vi "Periodic Tasks.vi"(8 "error in":errorcluster) -> ()   [LabVIEW 2020]
doc: "This VI runs in parallel to other tasks. It can contain as many user-defined periodic loops as you need. These can carry out PID or other sorts of timed response."
uses:
  <vilib>/Rock Robotics/WPI/ThirdParty/REV Robotics/REVLib/Typedef/Spark MAX Idle Mode.ctl
  <vilib>/Rock Robotics/WPI/DriverStation/WPI_DriverStationRobotMode2.ctl
  <vilib>/Rock Robotics/WPI/ThirdParty/JAS_Junk/TrajLib/LinearFilter_ResetToValue.vi
  <vilib>/Rock Robotics/WPI/ThirdParty/JAS_Junk/TrajLib/LinearFilter_Calculate.vi
  Robot Global Data.vi
  SUB VIs/TOGGLE GLOBAL.vi
  <vilib>/Rock Robotics/WPI/ThirdParty/JAS_Junk/TrajLib/LinearFilter_MovingAverage.vi
  <vilib>/Rock Robotics/WPI/ThirdParty/JAS_Junk/TrajLib/LinearFilter_LowPassBW1.vi
  <vilib>/Rock Robotics/WPI/ThirdParty/JAS_Junk/TrajLib/LinearFilter_LowPassBW2.vi
  <vilib>/Rock Robotics/WPI/ThirdParty/JAS_Junk/TrajLib/LinearFilter_HighPassBW1.vi
  <vilib>/Rock Robotics/WPI/ThirdParty/JAS_Junk/TrajLib/LinearFilter_HighPassBW2.vi
  <vilib>/Rock Robotics/WPI/ThirdParty/Phoenix-LabVIEW/Pigeon IMU/CTRE_PigeonIMU_GetYPR.vi
  <vilib>/Rock Robotics/WPI/Utilities/WPI_GetSetVariantRefNum.vi
  <vilib>/Rock Robotics/Network Tables/NT Read Number.vi
  <vilib>/Rock Robotics/Network Tables/NT Write Number.vi
  <vilib>/Rock Robotics/WPI/ThirdParty/JAS_Junk/TrajLib/Trajectory_Library.lvlib
  <vilib>/Rock Robotics/Network Tables/NT Write Boolean.vi
panel:
  in  "Idle Mode":T1
  in  "Output 4":dbl
  in  "Output 3":dbl
  in  "Output 1":dbl
  in  "Output 2":dbl
  out "CORRENTE ITK INF 2":dbl
  out "CORRENTE INTAKE 3":dbl(graph)
  out "DISTANCE ITK MVT SUP":dbl
  in  "RST MGVT SUP":bool
  in  "BREAK 3":bool
  in  "RST ITK 3":bool
  in  "AUX 14":bool
  in  "AUX 13":bool
  in  "AUX 12":bool
  in  "AUX 11":bool
  in  "AUX 10":bool
  in  "AUX 9":bool
  in  "AUX 8":bool
  in  "AUX 7":bool
  in  "AUX 6":bool
  in  "AUX 5":bool
  in  "AUX 3":dbl caption="LimeLight"
  in  "AUX 4":dbl caption="LimeLight"
  in  "AUX 2":dbl caption="LimeLight"
  in  "AUX 1":dbl caption="LimeLight"
  in  "Velocidade":dbl(slide) scale=0.0..1.0
  out "tx":dbl
  out "ty":dbl
  out "ta":dbl
  out "ts":dbl
  in  "RST ITK 2":bool
  out "DISTANCE CHASSI(m)":dbl
  in  "RST MECE":bool
  out "Yaw Pitch Roll":cluster{"Yaw":dbl, "Pitch":dbl, "Roll":dbl}={"Yaw"=0.5657958984375, "Pitch"=0.6591796875, "Roll"=0.0}
  out "DISTANCE ITK MVT":dbl
  in  "RST MGVT":bool
  out "CORRENTE ITK INF":dbl
  out "CORRENTE INTAKE 2":dbl(graph)
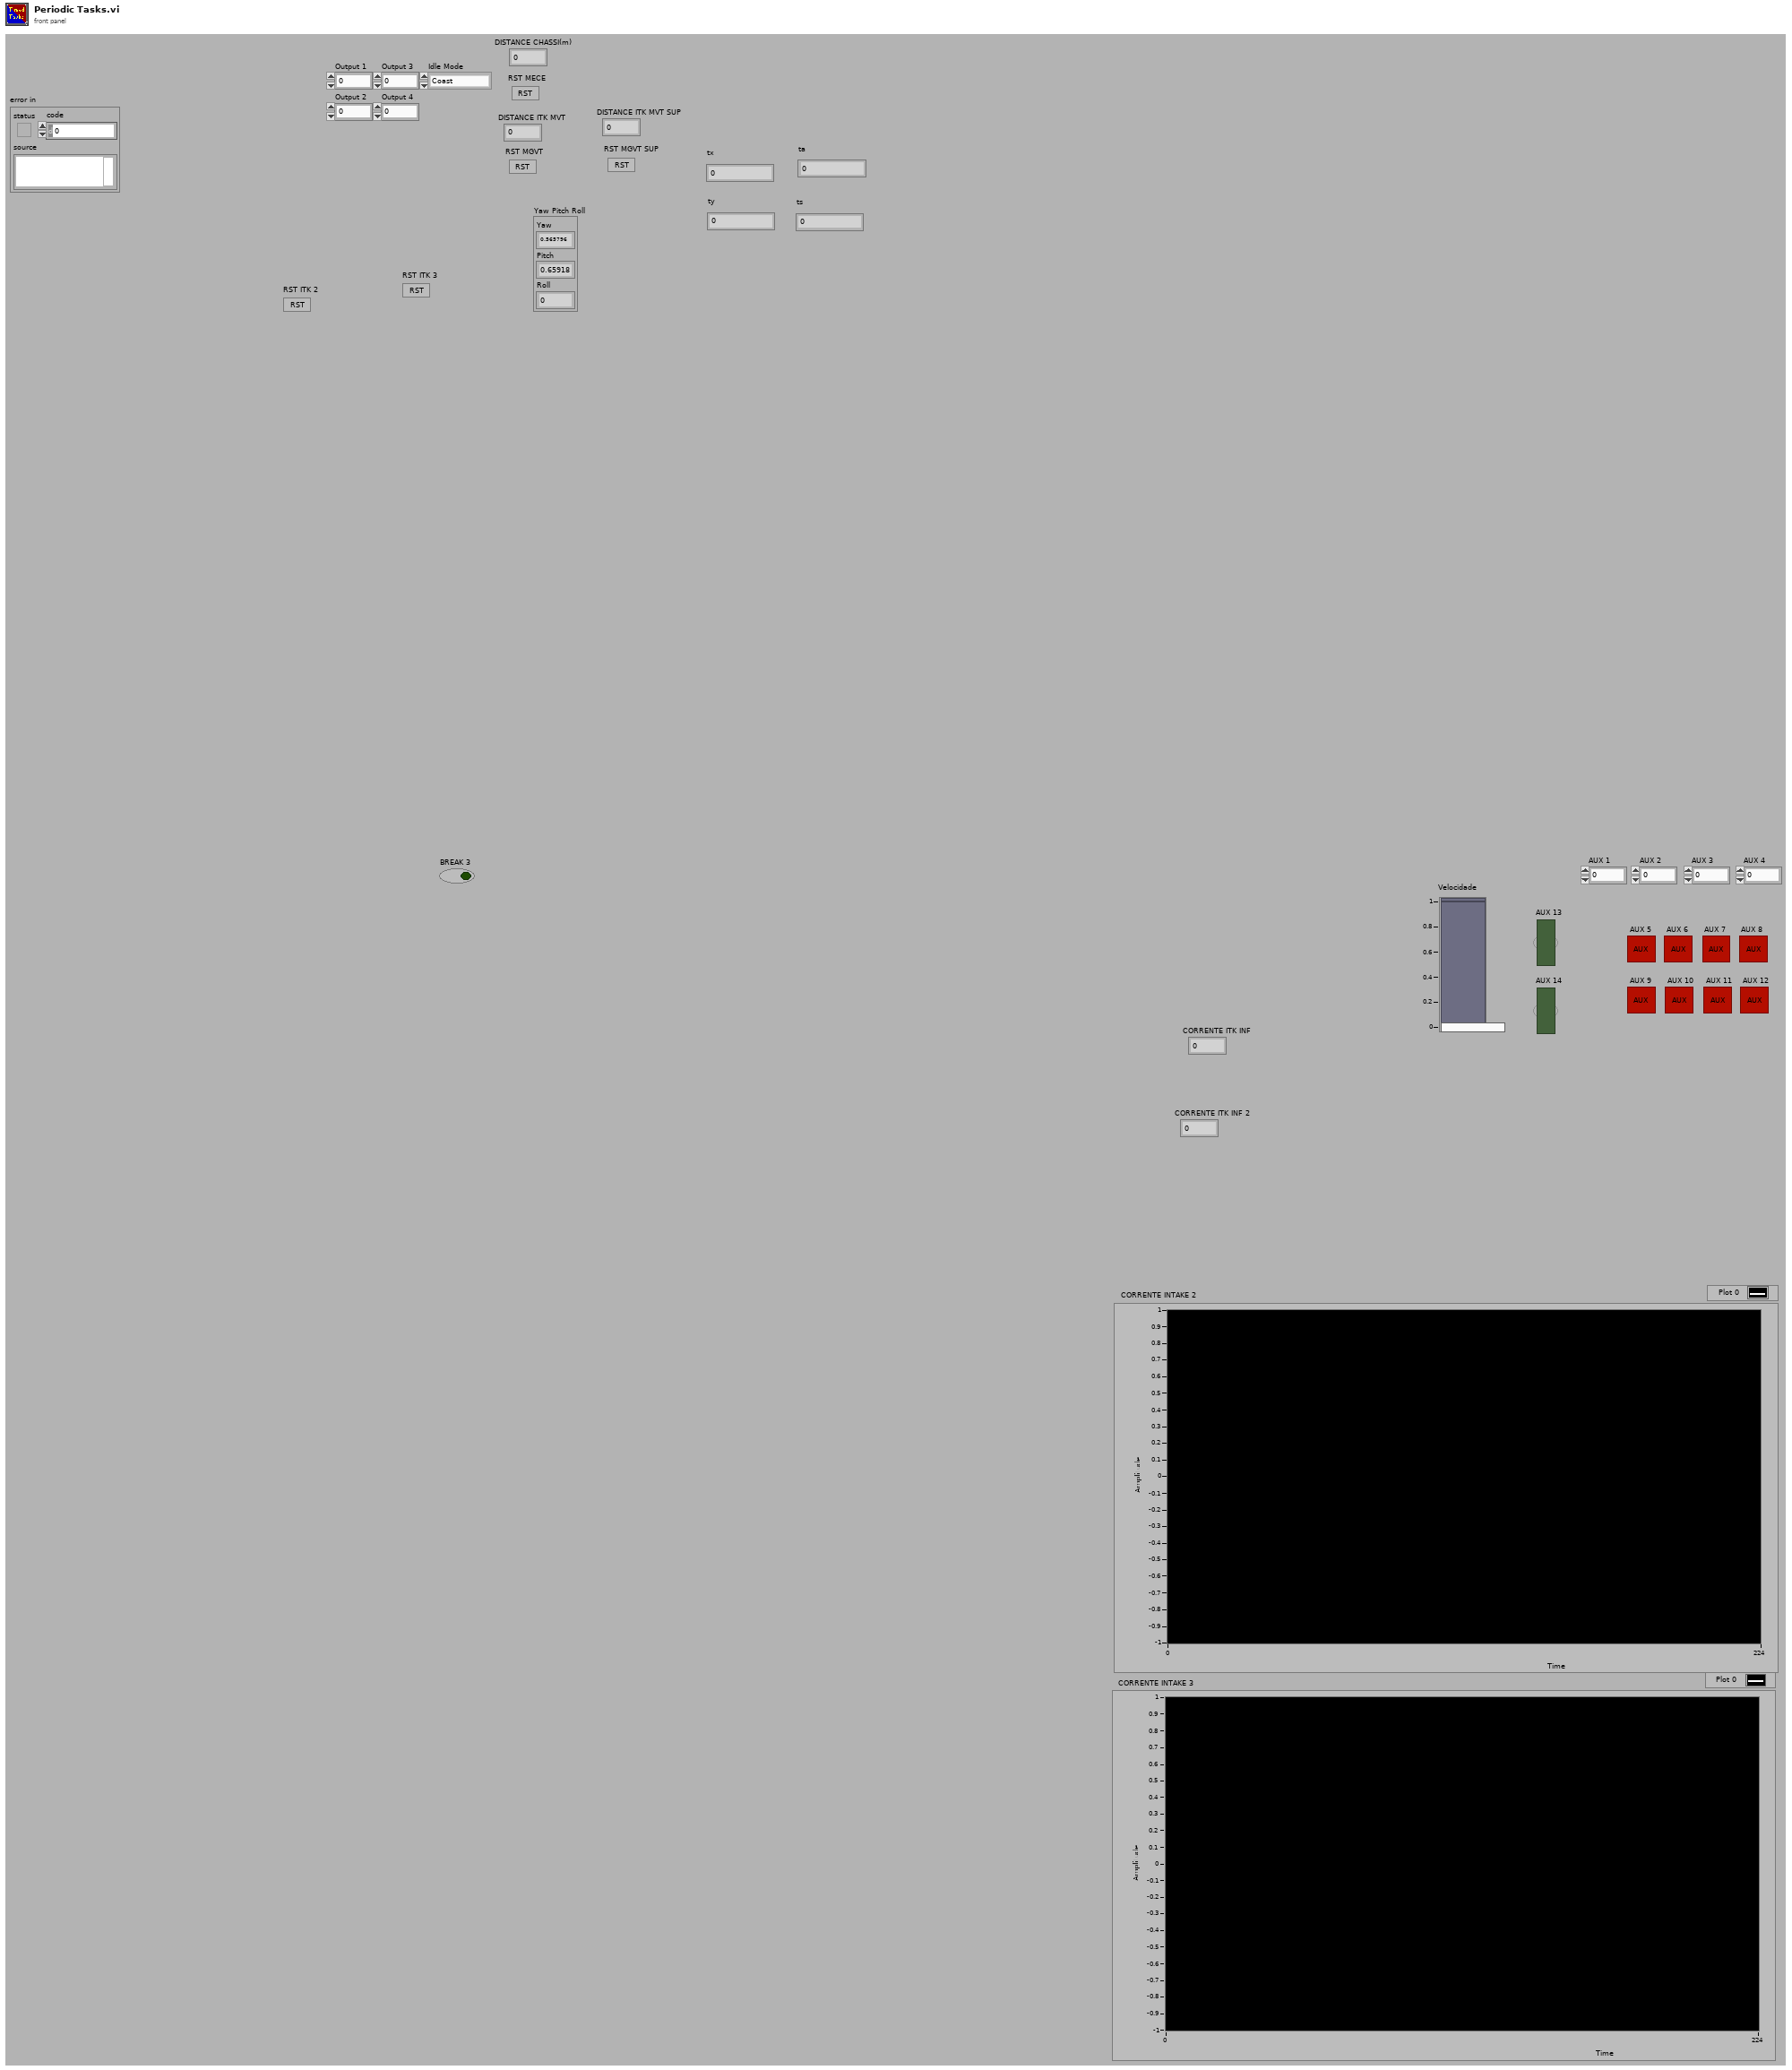
[diagram p1: front panel]
types:
  T1 = typedef "Spark MAX Idle Mode.ctl" = enum16{"Coast", "Brake"}
  T2 = typedef "WPI_MotorControlDeviceRef.ctl" = cluster{"DeviceStatus":errorcluster, "Type":T3, "PWM":cluster{"PWM Channel":T4, "DeadBand":T5}, "CAN":cluster{"Device Number":u8, "SetOutput VI Ref":variant, "GetOutput VI Ref":variant, "Enable VI Ref":variant, "Disable VI Ref":variant, "Data":variant}, "Invert":bool, "DIO PWM":cluster{"PWM \"Enable\" Channel":T4, "DIOChannel":T6, "PWM Rate":dbl}}
  T3 = typedef "WPI_MotorControlType.ctl" = enum16{"PWM", "CAN", "DIO PWM"}
  T4 = typedef "FPGA_DIOPWMChannel.ctl" = enum8{"PWM 0", "PWM 1", "PWM 2", "PWM 3", "PWM 4", "PWM 5", "PWM 6", "PWM 7", "PWM 8", "PWM 9", "PWM MXP 0", "PWM MXP 1", "PWM MXP 2", "PWM MXP 3", "PWM MXP 4", "PWM MXP 5", "PWM MXP 6", "PWM MXP 7", "PWM MXP 8", "PWM MXP 9", "Invalid"}
  T5 = typedef "WPI_PWMDeadband.ctl" = cluster{"Name":string, "maxPositivePwm":i32, "minPositivePwm":i32, "centerPwm":i32, "maxNegativePwm":i32, "minNegativePwm":i32, "angularRange":u16}
  T6 = typedef "FPGA_DIOChannel.ctl" = enum8{"DIO 0", "DIO 1", "DIO 2", "DIO 3", "DIO 4", "DIO 5", "DIO 6", "DIO 7", "DIO 8", "DIO 9", "DIO MXP 0", "DIO MXP 1", "DIO MXP 2", "DIO MXP 3", "DIO MXP 4", "DIO MXP 5", "DIO MXP 6", "DIO MXP 7", "DIO MXP 8", "DIO MXP 9", "DIO MXP 10", "DIO MXP 11", "DIO MXP 12", "DIO MXP 13", "DIO MXP 14", "DIO MXP 15", "SPI Port CS1", "SPI Port CS2", "SPI Port CS3", "SPI Port MISO", "SPI Port MOSI", "Invalid"}
  T7 = typedef "WPI_ServoDeviceRef.ctl" = cluster{"DeviceStatus":errorcluster, "PWM Channel":T4, "DeadBand":T5}
  T8 = typedef "WPI_JoystickDevRef.ctl" = cluster{"Device":T9}
  T9 = typedef "WPI_JoystickDeviceEnum.ctl" = enum16{"USB 0", "USB 1", "USB 2", "USB 3", "USB 4", "USB 5"}
  T10 = typedef "WPI_DigitalInputDevRef.ctl" = cluster{"DevStatus":errorcluster, "DIO Channel":T6}
  T11 = typedef "WPI_EncoderDevRef.ctl" = cluster{"DevStatus":errorcluster, "EncoderIndex":T12, "CounterIndex":T13, "DistancePerCount":dbl, "Decoding Type":T14}
  T12 = typedef "FPGA_EncoderIdx.ctl" = enum8{"Enc 0", "Enc 1", "Enc 2", "Enc 3", "Enc 4", "Enc 5", "Enc 6", "Enc 7", "Invalid"}
  T13 = typedef "FPGA_CounterCtrSystemIndex.ctl" = enum8{"Ctr 0", "Ctr 1", "Ctr 2", "Ctr 3", "Ctr 4", "Ctr 5", "Ctr 6", "Ctr 7", "Invalid"}
  T14 = typedef "WPI_EncoderType.ctl" = enum16{"1x", "2x", "4x"}
  T15 = typedef "CTRE_PigeonIMU_DeviceRef.ctl" = cluster{"DeviceStatus":errorcluster, "Device Number":u8, "Type":T16, "Device ID":u32, "Handle":u64, "UsageFrame":u32, "Library Path":path}
  T16 = typedef "CTRE_PigeonIMU_ConnectionType.ctl" = u32
  T17 = enum16{"Moving Average", "Low Pass 1st Order Butterworth", "Low Pass 2nd Order Butterworth", "High Pass 1st Order Butterworth", "High Pass 2nd Order Butterworth"}
  T18 = typedef "WPI_DriverStationRobotMode2.ctl" = enum16{"Autonomous Disabled", "Autonomous Enabled", "Teleop Disabled", "Teleop Enabled", "Disconnected", "Finish", "Test Disabled", "Test Enabled", "Emergency Stopped"}
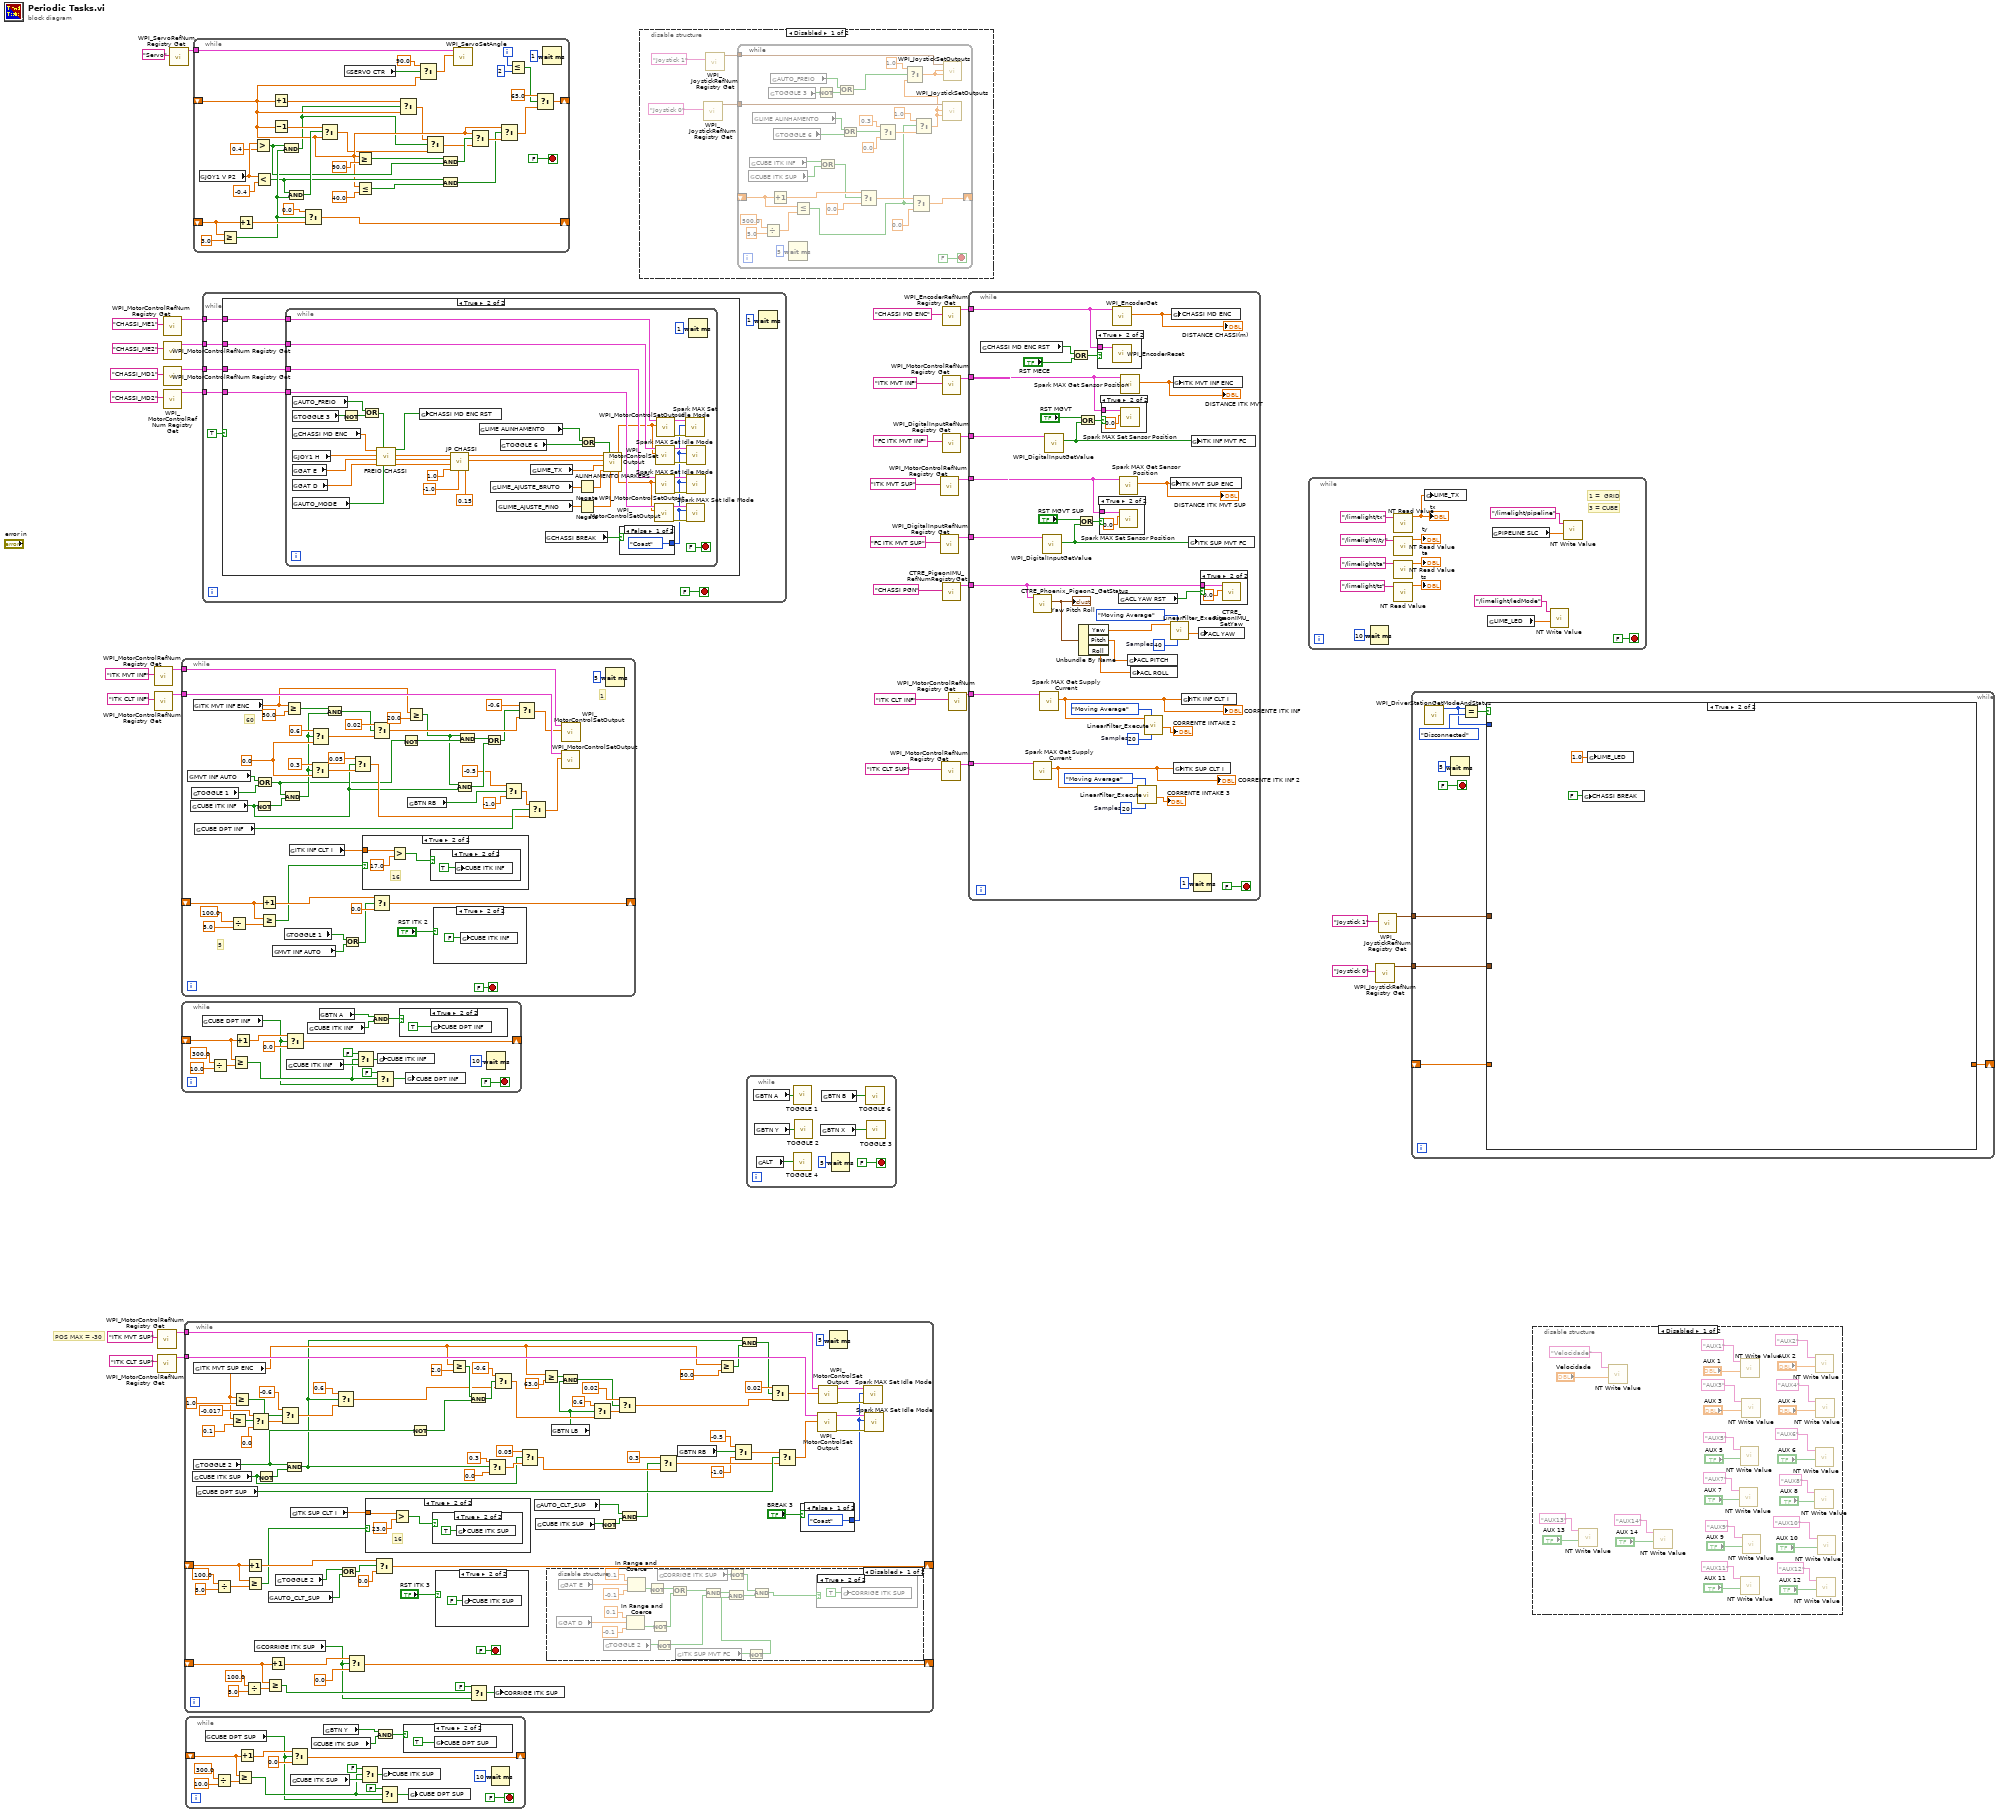
[diagram p0: block diagram]
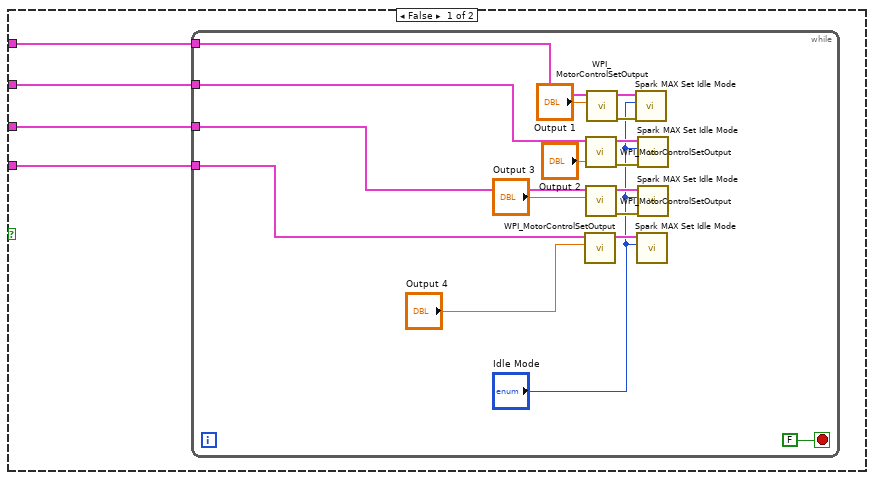
[diagram p2: hidden frame]
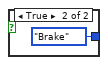
[diagram p3: hidden frame]
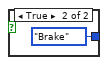
[diagram p11: hidden frame]
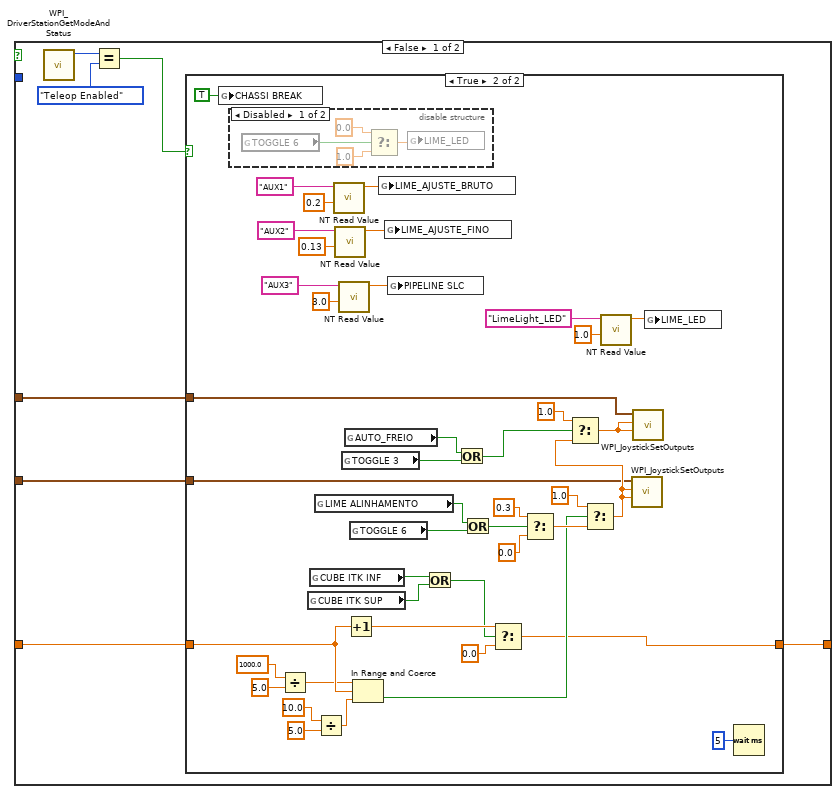
[diagram p13: hidden frame]
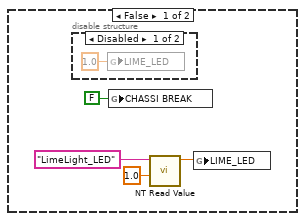
[diagram p14: hidden frame]
diagram:
  # "POS MAX = -30"
  n1 = call <vilib>:"WPI_MotorControlRefNum Registry Get.vi"("refnum name"="ITK MVT INF") -> ("MotorControlDevRef"=w29:T2)  [unwired: 9 in, 1 out]
  n2 = call <vilib>:"WPI_MotorControlRefNum Registry Get.vi"("refnum name"="ITK CLT INF") -> ("MotorControlDevRef"=w27:T2)  [unwired: 9 in, 1 out]
  n3 = call <vilib>:"WPI_MotorControlRefNum Registry Get.vi"("refnum name"="ITK MVT SUP") -> ("MotorControlDevRef"=w14:T2)  [unwired: 9 in, 1 out]
  n4 = call <vilib>:"WPI_MotorControlRefNum Registry Get.vi"("refnum name"="ITK CLT SUP") -> ("MotorControlDevRef"=w13:T2)  [unwired: 9 in, 1 out]
  n5 = call <vilib>:"WPI_MotorControlRefNum Registry Get.vi"("refnum name"="CHASSI_ME1") -> ("MotorControlDevRef"=w37:T2)  [unwired: 9 in, 1 out]
  n6 = call <vilib>:"WPI_MotorControlRefNum Registry Get.vi"("refnum name"="CHASSI_ME2") -> ("MotorControlDevRef"=w33:T2)  [unwired: 9 in, 1 out]
  n7 = call <vilib>:"WPI_MotorControlRefNum Registry Get.vi"("refnum name"="CHASSI_MD1") -> ("MotorControlDevRef"=w32:T2)  [unwired: 9 in, 1 out]
  n8 = call <vilib>:"WPI_MotorControlRefNum Registry Get.vi"("refnum name"="CHASSI_MD2") -> ("MotorControlDevRef"=w31:T2)  [unwired: 9 in, 1 out]
  n9 = call <vilib>:"WPI_ServoRefNum Registry Get.vi"("refnum name"="Servo") -> ("ServoDeviceRef"=w5:T7)  [unwired: 9 in, 1 out]
  n10 = while {
    tunnel: w29 -> [w87]
    tunnel: w27 -> [w86]
    shift-right: [w75] -> _
    shift-left: _ -> [w74]
    stop <- FALSE stop-if-true
    w82 = 0.0 ("Output")
    # "60"
    # "5"
    # "1"
    n11 = global read "Robot Global Data.vi" "MVT INF AUTO"() -> (w46:bool)
    n12 = global read "Robot Global Data.vi" "CUBE ITK INF"() -> (w53:bool)
    n13 = global read "TOGGLE GLOBAL.vi" "TOGGLE 1"() -> (w47:bool)
    n14 = global read "Robot Global Data.vi" "ITK MVT INF ENC"() -> (w50:dbl)
    n15 = global read "Robot Global Data.vi" "CUBE DPT INF"() -> (w69:bool)
    n16 = Divide(x=100.0, y=5.0) -> (x/y=w79:dbl)
    n17 = Not(x=w53) -> (.not. x?=w71:bool)
    n18 = Or(x=w46, y=w47) -> (x .or. y?=w48:bool)
    n19 = Increment(x=w74) -> (x+1=w81:dbl)
    n20 = Greater Or Equal?(x=w74, y=w79) -> (x >= y?=w72:bool)
    n21 = global read "Robot Global Data.vi" "MVT INF AUTO"() -> (w45:bool)
    n22 = And(x=w48, y=w71) -> (x .and. y?=w60:bool)
    n23 = global read "TOGGLE GLOBAL.vi" "TOGGLE 1"() -> (w44:bool)
    n24 = Greater Or Equal?(x=w50, y=50.0) -> (x >= y?=w62:bool)
    n25 = global read "Robot Global Data.vi" "ITK INF CLT I"() -> (w73:dbl)
    n26 = Select(t=0.3, s=w60, f=w82) -> (s? t:f=w68:dbl)
    n27 = Select(t=0.6, s=w60, f=w82) -> (s? t:f=w65:dbl)
    n28 = And(x=w62, y=w60) -> (x .and. y?=w61:bool)
    n29 = Or(x=w44, y=w45) -> (x .or. y?=w43:bool)
    n30 = Select(t=0.05, s=w53, f=w68) -> (s? t:f=w67:dbl)
    n31 = case shown="True" w72 {
      tunnel: w73 -> [_ w91]
      frame False {
      }
      frame True {
        # "16"
        n32 = Greater?(x=w91, y=17.0) -> (0:w89:bool)
        n33 = case shown="True" w89 {
          frame False {
          }
          frame True {
            n34 = global write "Robot Global Data.vi" "CUBE ITK INF"(TRUE ("CONE ITK")) -> ()
          }
        }
      }
    }
    n35 = Select(t=0.02, s=w61, f=w65) -> (s? t:f=w57:dbl)
    n36 = Select(t=w81, s=w43, f=0.0) -> (s? t:f=w75:dbl)
    n37 = Not(x=w48) -> (.not. x?=w56:bool)
    n38 = Greater Or Equal?(x=w50, y=20.0) -> (x >= y?=w52:bool)
    n39 = global read "Robot Global Data.vi" "BTN RB"() -> (w39:bool)
    n40 = case shown="True" "RST ITK 2" {
      frame False {
      }
      frame True {
        n41 = global write "Robot Global Data.vi" "CUBE ITK INF"(FALSE ("CONE ITK")) -> ()
      }
    }
    n42 = And(x=w52, y=w53) -> (x .and. y?=w51:bool)
    n43 = And(x=w52, y=w56) -> (x .and. y?=w55:bool)
    n44 = Or(x=w55, y=w51) -> (x .or. y?=w54:bool)
    n45 = Select(t=-0.5, s=w39, f=-1.0 ("t")) -> (s? t:f=w42:dbl)
    n46 = Select(t=-0.6, s=w54, f=w57) -> (s? t:f=w49:dbl)
    n47 = Select(t=w42, s=w69, f=w67) -> (s? t:f=w70:dbl)
    n48 = call <vilib>:"WPI_MotorControlSetOutput.vi"("Output"=w70, "MotorControlDevRef"=w86) -> ()  [unwired: 7 in, 3 out]
    n49 = call <vilib>:"WPI_MotorControlSetOutput.vi"("Output"=w49, "MotorControlDevRef"=w87) -> ()  [unwired: 7 in, 3 out]
    n50 = Wait (ms)(milliseconds to wait=u32 5) -> ()  [unwired: 1 out]
  }
  n51 = while {
    shift-right: [w105] -> _
    shift-left: _ -> [w110]
    stop <- FALSE stop-if-true
    n52 = global read "Robot Global Data.vi" "CUBE DPT INF"() -> (w94:bool)
    n53 = Divide(x=300.0, y=10.0) -> (x/y=w111:dbl)
    n54 = Greater Or Equal?(x=w110, y=w111) -> (x >= y?=w95:bool)
    n55 = Increment(x=w110) -> (x+1=w106:dbl)
    n56 = Select(t=w106, s=w94, f=0.0) -> (s? t:f=w105:dbl)
    n57 = global read "Robot Global Data.vi" "CUBE ITK INF"() -> (w101:bool)
    n58 = global read "Robot Global Data.vi" "CUBE ITK INF"() -> (w99:bool)
    n59 = global read "Robot Global Data.vi" "BTN A"() -> (w98:bool)
    n60 = Select(t=FALSE, s=w95, f=w101) -> (s? t:f=w103:bool)
    n61 = And(x=w98, y=w99) -> (x .and. y?=w100:bool)
    n62 = Select(t=FALSE, s=w95, f=w94) -> (s? t:f=w96:bool)
    n63 = global write "Robot Global Data.vi" "CUBE ITK INF"(w103) -> ()
    n64 = case shown="True" w100 {
      frame False {
      }
      frame True {
        n65 = global write "Robot Global Data.vi" "CUBE DPT INF"(TRUE ("BTN5")) -> ()
      }
    }
    n66 = global write "Robot Global Data.vi" "CUBE DPT INF"(w96) -> ()
    n67 = Wait (ms)(milliseconds to wait=u32 10) -> ()  [unwired: 1 out]
  }
  n68 = while {
    tunnel: w14 -> [w198]
    tunnel: w13 -> [w197]
    shift-right: [w180] -> _
    shift-left: _ -> [w179]
    shift-right: [w133] -> _
    shift-left: _ -> [w134]
    stop <- FALSE stop-if-true
    n69 = global read "Robot Global Data.vi" "CUBE ITK SUP"() -> (w171:bool)
    n70 = global read "Robot Global Data.vi" "ITK MVT SUP ENC"() -> (w124:dbl)
    n71 = global read "TOGGLE GLOBAL.vi" "TOGGLE 2"() -> (w170:bool)
    n72 = global read "Robot Global Data.vi" "CUBE DPT SUP"() -> (w174:bool)
    n73 = Divide(x=100.0, y=5.0) -> (x/y=w184:dbl)
    n74 = Greater Or Equal?(x=w124, y=0.1) -> (x >= y?=w150:bool)
    n75 = Greater Or Equal?(x=w124, y=1.0) -> (x >= y?=w162:bool)
    n76 = Divide(x=100.0, y=5.0) -> (x/y=w135:dbl)
    n77 = Increment(x=w179) -> (x+1=w186:dbl)
    n78 = Greater Or Equal?(x=w179, y=w184) -> (x >= y?=w177:bool)
    n79 = Select(t=-0.017, s=w150, f=0.0) -> (s? t:f=w165:dbl)
    n80 = global read "Robot Global Data.vi" "CORRIGE ITK SUP"() -> (w127:bool)
    n81 = Not(x=w171) -> (.not. x?=w176:bool)
    n82 = Greater Or Equal?(x=w134, y=w135) -> (x >= y?=w128:bool)
    n83 = global read "Robot Global Data.vi" "AUTO_CLT_SUP"() -> (w145:bool)
    n84 = Increment(x=w134) -> (x+1=w132:dbl)
    n85 = global read "TOGGLE GLOBAL.vi" "TOGGLE 2"() -> (w146:bool)
    n86 = Select(t=-0.6, s=w162, f=w165) -> (s? t:f=w166:dbl)
    n87 = And(x=w170, y=w176) -> (x .and. y?=w115:bool)
    n88 = global read "Robot Global Data.vi" "ITK SUP CLT I"() -> (w178:dbl)
    n89 = Select(t=0.6, s=w115, f=w166) -> (s? t:f=w120:dbl)
    n90 = Or(x=w146, y=w145) -> (x .or. y?=w147:bool)
    n91 = Select(t=w132, s=w127, f=0.0) -> (s? t:f=w133:dbl)
    n92 = case shown="True" w177 {
      tunnel: w178 -> [_ w223]
      frame False {
      }
      frame True {
        # "16"
        n93 = Greater?(x=w223, y=23.0) -> (0:w221:bool)
        n94 = case shown="True" w221 {
          frame False {
          }
          frame True {
            n95 = global write "Robot Global Data.vi" "CUBE ITK SUP"(TRUE ("CONE ITK")) -> ()
          }
        }
      }
    }
    n96 = Select(t=w186, s=w147, f=0.0) -> (s? t:f=w180:dbl)
    n97 = Not(x=w170) -> (.not. x?=w148:bool)
    n98 = case shown="True" "RST ITK 3" {
      frame False {
      }
      frame True {
        n99 = global write "Robot Global Data.vi" "CUBE ITK SUP"(FALSE ("CONE ITK")) -> ()
      }
    }
    n100 = Greater Or Equal?(x=w124, y=2.0) -> (x >= y?=w161:bool)
    n101 = And(x=w161, y=w148) -> (x .and. y?=w160:bool)
    n102 = Select(t=FALSE, s=w128, f=w127) -> (s? t:f=w130:bool)
    n103 = Select(t=0.3, s=w115, f=0.0 ("Output")) -> (s? t:f=w173:dbl)
    n104 = Select(t=-0.6, s=w160, f=w120) -> (s? t:f=w155:dbl)
    n105 = global write "Robot Global Data.vi" "CORRIGE ITK SUP"(w130) -> ()
    n106 = Select(t=0.05, s=w171, f=w173) -> (s? t:f=w143:dbl)
    n107 = global read "Robot Global Data.vi" "AUTO_CLT_SUP"() -> (w140:bool)
    n108 = global read "Robot Global Data.vi" "CUBE ITK SUP"() -> (w142:bool)
    n109 = Greater Or Equal?(x=w124, y=63.0) -> (x >= y?=w154:bool)
    n110 = disable-structure shown="Disabled" {
      frame Disabled {
        n111 = global read "Robot Global Data.vi" "GAT D"() -> (w214:dbl)
        n112 = global read "Robot Global Data.vi" "GAT E"() -> (w219:dbl)
        n113 = global read "TOGGLE GLOBAL.vi" "TOGGLE 2"() -> (w208:bool)
        n114 = In Range and Coerce(upper limit=0.1, x=w214, lower limit=-0.1) -> (In Range?=w211:bool)  [unwired: 1 out]
        n115 = In Range and Coerce(upper limit=0.1, x=w219, lower limit=-0.1) -> (In Range?=w213:bool)  [unwired: 1 out]
        n116 = Not(x=w213) -> (.not. x?=w212:bool)
        n117 = Not(x=w211) -> (.not. x?=w210:bool)
        n118 = Not(x=w208) -> (.not. x?=w207:bool)
        n119 = global read "Robot Global Data.vi" "CORRIGE ITK SUP"() -> (w202:bool)
        n120 = Or(x=w212, y=w210) -> (x .or. y?=w209:bool)
        n121 = global read "Robot Global Data.vi" "ITK SUP MVT FC"() -> (w206:bool)
        n122 = And(x=w209, y=w207) -> (x .and. y?=w203:bool)
        n123 = Not(x=w202) -> (.not. x?=w201:bool)
        n124 = Not(x=w206) -> (.not. x?=w205:bool)
        n125 = And(x=w203, y=w205) -> (x .and. y?=w204:bool)
        n126 = And(x=w201, y=w204) -> (x .and. y?=w200:bool)
        n127 = case shown="True" w200 {
          frame False {
          }
          frame True {
            n128 = global write "Robot Global Data.vi" "CORRIGE ITK SUP"(TRUE ("CORRIGE ITK SUP")) -> ()
          }
        }
      }
      frame Enabled {
      }
    }
    n129 = global read "Robot Global Data.vi" "BTN LB"() -> (w152:bool)
    n130 = And(x=w154, y=w152) -> (x .and. y?=w153:bool)
    n131 = Select(t=0.6, s=w152, f=w155) -> (s? t:f=w157:dbl)
    n132 = Not(x=w142) -> (.not. x?=w141:bool)
    n133 = Select(t=0.02, s=w153, f=w157) -> (s? t:f=w114:dbl)
    n134 = And(x=w140, y=w141) -> (x .and. y?=w139:bool)
    n135 = Select(t=0.3, s=w139, f=w143) -> (s? t:f=w144:dbl)
    n136 = global read "Robot Global Data.vi" "BTN RB"() -> (w116:bool)
    n137 = Greater Or Equal?(x=w124, y=50.0) -> (x >= y?=w123:bool)
    n138 = Select(t=-0.5, s=w116, f=-1.0 ("t")) -> (s? t:f=w119:dbl)
    n139 = And(x=w115, y=w123) -> (x .and. y?=w121:bool)
    n140 = Select(t=0.02, s=w121, f=w114) -> (s? t:f=w126:dbl)
    n141 = Select(t=w119, s=w174, f=w144) -> (s? t:f=w175:dbl)
    n142 = case shown="False" "BREAK 3" {
      tunnel: [Spark_MAX_Idle_Mode."Coast" ("Idle Mode") Spark_MAX_Idle_Mode."Brake" ("Idle Mode")] -> w190
      frame False {
      }
      frame True {
      }
    }
    n143 = call <vilib>:"WPI_MotorControlSetOutput.vi"("Output"=w175, "MotorControlDevRef"=w197) -> ("error out"=w192:errorcluster, "MotorControlDevRef"=w193:T2)  [unwired: 7 in, 1 out]
    n144 = call <vilib>:"WPI_MotorControlSetOutput.vi"("Output"=w126, "MotorControlDevRef"=w198) -> ("error out"=w194:errorcluster, "MotorControlDevRef"=w195:T2)  [unwired: 7 in, 1 out]
    n145 = Wait (ms)(milliseconds to wait=u32 5) -> ()  [unwired: 1 out]
    n146 = call <vilib>:"Spark MAX Set Idle Mode.vi"("error in (no error)"=w194, "Idle Mode"=w190, "MotorControlDeviceRef in"=w195) -> ()  [unwired: 7 in, 2 out]
    n147 = call <vilib>:"Spark MAX Set Idle Mode.vi"("error in (no error)"=w192, "Idle Mode"=w190, "MotorControlDeviceRef in"=w193) -> ()  [unwired: 7 in, 2 out]
  }
  n148 = while {
    shift-right: [w239] -> _
    shift-left: _ -> [w244]
    stop <- FALSE stop-if-true
    n149 = global read "Robot Global Data.vi" "CUBE DPT SUP"() -> (w228:bool)
    n150 = Divide(x=300.0, y=10.0) -> (x/y=w245:dbl)
    n151 = Greater Or Equal?(x=w244, y=w245) -> (x >= y?=w229:bool)
    n152 = Increment(x=w244) -> (x+1=w240:dbl)
    n153 = Select(t=w240, s=w228, f=0.0) -> (s? t:f=w239:dbl)
    n154 = global read "Robot Global Data.vi" "CUBE ITK SUP"() -> (w235:bool)
    n155 = global read "Robot Global Data.vi" "CUBE ITK SUP"() -> (w233:bool)
    n156 = global read "Robot Global Data.vi" "BTN Y"() -> (w232:bool)
    n157 = Select(t=FALSE, s=w229, f=w235) -> (s? t:f=w237:bool)
    n158 = And(x=w232, y=w233) -> (x .and. y?=w234:bool)
    n159 = Select(t=FALSE, s=w229, f=w228) -> (s? t:f=w230:bool)
    n160 = global write "Robot Global Data.vi" "CUBE ITK SUP"(w237) -> ()
    n161 = case shown="True" w234 {
      frame False {
      }
      frame True {
        n162 = global write "Robot Global Data.vi" "CUBE DPT SUP"(TRUE ("BTN5")) -> ()
      }
    }
    n163 = global write "Robot Global Data.vi" "CUBE DPT SUP"(w230) -> ()
    n164 = Wait (ms)(milliseconds to wait=u32 10) -> ()  [unwired: 1 out]
  }
  n165 = while {
    shift-right: [w281] -> _
    shift-left: _ -> [w283]
    shift-right: [w273] -> _
    shift-left: _ -> [w251]
    tunnel: w5 -> [w256]
    i -> [w272]
    stop <- FALSE stop-if-true
    n166 = global read "Robot Global Data.vi" "JOY1 V P2"() -> (w276:dbl)
    n167 = Greater Or Equal?(x=w283, y=3.0) -> (x >= y?=w260:bool)
    n168 = Increment(x=w283) -> (x+1=w280:dbl)
    n169 = Greater?(x=w276, y=0.4) -> (0:w259:bool)
    n170 = Less?(x=w276, y=-0.4 ("x")) -> (x < y?=w257:bool)
    n171 = Increment(x=w251) -> (x+1=w278:dbl)
    n172 = Decrement(x=w251) -> (x-1=w274:dbl)
    n173 = And(x=w259, y=w260) -> (x .and. y?=w249:bool)
    n174 = And(x=w257, y=w260) -> (x .and. y?=w261:bool)
    n175 = Select(t=0.0 ("f"), s=w260, f=w280) -> (s? t:f=w281:dbl)
    n176 = Select(t=w274, s=w261, f=w251) -> (s? t:f=w250:dbl)
    n177 = global read "Robot Global Data.vi" "SERVO CTR"() -> (w254:bool)
    n178 = Greater Or Equal?(x=w251, y=90.0) -> (x >= y?=w264:bool)
    n179 = Less Or Equal?(x=w251, y=40.0) -> (x <= y?=w258:bool)
    n180 = Select(t=w278, s=w249, f=w251) -> (s? t:f=w248:dbl)
    n181 = Select(t=90.0, s=w254, f=w251) -> (s? t:f=w255:dbl)
    n182 = Select(t=w248, s=w249, f=w250) -> (s? t:f=w252:dbl)
    n183 = And(x=w264, y=w259) -> (x .and. y?=w262:bool)
    n184 = And(x=w257, y=w258) -> (x .and. y?=w263:bool)
    n185 = call <vilib>:"WPI_ServoSetAngle.vi"("Angle"=w255, "ServoDeviceRef"=w256) -> ()  [unwired: 8 in, 2 out]
    n186 = Select(t=w251, s=w262, f=w252) -> (s? t:f=w266:dbl)
    n187 = Select(t=w251, s=w263, f=w266) -> (s? t:f=w267:dbl)
    n188 = Less Or Equal?(x=w272, y=2) -> (x <= y?=w269:bool)
    n189 = Select(t=65.0, s=w269, f=w267) -> (s? t:f=w273:dbl)
    n190 = Wait (ms)(milliseconds to wait=u32 1) -> ()  [unwired: 1 out]
  }
  n191 = while {
    tunnel: w37 -> [w292]
    tunnel: w33 -> [w291]
    tunnel: w32 -> [w290]
    tunnel: w31 -> [w289]
    stop <- FALSE stop-if-true
    n192 = case shown="True" TRUE {
      tunnel: w292 -> [w296 w317]
      tunnel: w291 -> [w295 w316]
      tunnel: w290 -> [w294 w315]
      tunnel: w289 -> [w293 w314]
      frame False {
        n193 = while {
          tunnel: w296 -> [w305]
          tunnel: w295 -> [w304]
          tunnel: w294 -> [w303]
          tunnel: w293 -> [w302]
          stop <- FALSE stop-if-true
          n194 = call <vilib>:"WPI_MotorControlSetOutput.vi"("Output"="Output 4", "MotorControlDevRef"=w302) -> ("MotorControlDevRef"=w307:T2)  [unwired: 7 in, 2 out]
          n195 = call <vilib>:"WPI_MotorControlSetOutput.vi"("Output"="Output 2", "MotorControlDevRef"=w304) -> ("error out"=w310:errorcluster, "MotorControlDevRef"=w311:T2)  [unwired: 7 in, 1 out]
          n196 = call <vilib>:"WPI_MotorControlSetOutput.vi"("Output"="Output 3", "MotorControlDevRef"=w303) -> ("error out"=w308:errorcluster, "MotorControlDevRef"=w309:T2)  [unwired: 7 in, 1 out]
          n197 = call <vilib>:"WPI_MotorControlSetOutput.vi"("Output"="Output 1", "MotorControlDevRef"=w305) -> ("error out"=w312:errorcluster, "MotorControlDevRef"=w313:T2)  [unwired: 7 in, 1 out]
          n198 = call <vilib>:"Spark MAX Set Idle Mode.vi"("error in (no error)"=w312, "Idle Mode"="Idle Mode", "MotorControlDeviceRef in"=w313) -> ()  [unwired: 7 in, 2 out]
          n199 = call <vilib>:"Spark MAX Set Idle Mode.vi"("Idle Mode"="Idle Mode", "MotorControlDeviceRef in"=w307) -> ()  [unwired: 8 in, 2 out]
          n200 = call <vilib>:"Spark MAX Set Idle Mode.vi"("error in (no error)"=w310, "Idle Mode"="Idle Mode", "MotorControlDeviceRef in"=w311) -> ()  [unwired: 7 in, 2 out]
          n201 = call <vilib>:"Spark MAX Set Idle Mode.vi"("error in (no error)"=w308, "Idle Mode"="Idle Mode", "MotorControlDeviceRef in"=w309) -> ()  [unwired: 7 in, 2 out]
        }
      }
      frame True {
        n202 = while {
          tunnel: w317 -> [w358]
          tunnel: w316 -> [w357]
          tunnel: w315 -> [w356]
          tunnel: w314 -> [w355]
          stop <- FALSE stop-if-true
          n203 = global read "Robot Global Data.vi" "AUTO_FREIO"() -> (w320:bool)
          n204 = global read "TOGGLE GLOBAL.vi" "TOGGLE 3"() -> (w324:bool)
          n205 = global read "Robot Global Data.vi" "CHASSI MD ENC"() -> (w325:dbl)
          n206 = global read "Robot Global Data.vi" "JOY1 H"() -> (w331:dbl)
          n207 = global read "Robot Global Data.vi" "GAT E"() -> (w330:dbl)
          n208 = global read "Robot Global Data.vi" "GAT D"() -> (w329:dbl)
          n209 = global read "Robot Global Data.vi" "AUTO_MODE"() -> (w319:bool)
          n210 = Not(x=w324) -> (.not. x?=w321:bool)
          n211 = Or(x=w320, y=w321) -> (x .or. y?=w322:bool)
          n212 = call "FREIO CHASSI.vi"("MODE  T/A"=w319, "ENABLE"=w322, "IN Axes3"=w329, "IN Axes2"=w330, "IN Axes0"=w331, "IN ENC"=w325) -> ("OUT Axes3"=w327:dbl, "OUT Axes2"=w326:dbl, "OUT Axes0"=w328:dbl, "RST ENC"=w323:bool)
          n213 = global write "Robot Global Data.vi" "CHASSI MD ENC RST"(w323) -> ()
          n214 = call "JP CHASSI.vi"("In Axes 0"=w328, "In Axes 2"=w326, "In Axes 3"=w327, "POV In"=-1.0 ("t"), "In Dashboard"=1.0, "V Motor POV"=0.15) -> ("MESQ OUT"=w344:dbl, "MDIR OUT"=w343:dbl)  [unwired: 1 in]
          n215 = global read "Robot Global Data.vi" "LIME ALINHAMENTO"() -> (w332:bool)
          n216 = global read "Robot Global Data.vi" "LIME_AJUSTE_BRUTO"() -> (w335:dbl)
          n217 = global read "Robot Global Data.vi" "LIME_AJUSTE_FINO"() -> (w337:dbl)
          n218 = global read "TOGGLE GLOBAL.vi" "TOGGLE 6"() -> (w333:bool)
          n219 = global read "Robot Global Data.vi" "LIME_TX"() -> (w340:dbl)
          n220 = global read "Robot Global Data.vi" "CHASSI BREAK"() -> (w339:bool)
          n221 = Negate(x=w335) -> (-x=w336:dbl)
          n222 = Negate(x=w337) -> (-x=w338:dbl)
          n223 = Or(x=w332, y=w333) -> (x .or. y?=w334:bool)
          n224 = call "ALINHAMENTO MARKERS.vi"("MESQ IN"=w344, "EN"=w334, "MDIR IN"=w343, "TX MARKER"=w340, "V_Fina"=w338, "V_Bruta"=w336) -> ("MESQ OUT"=w342:dbl, "MDIR OUT"=w341:dbl)  [unwired: 1 in]
          n225 = case shown="False" w339 {
            tunnel: [Spark_MAX_Idle_Mode."Coast" ("Idle Mode") Spark_MAX_Idle_Mode."Brake" ("Idle Mode")] -> w345
            frame False {
            }
            frame True {
            }
          }
          n226 = call <vilib>:"WPI_MotorControlSetOutput.vi"("Output"=w341, "MotorControlDevRef"=w355) -> ("error out"=w346:errorcluster, "MotorControlDevRef"=w347:T2)  [unwired: 7 in, 1 out]
          n227 = call <vilib>:"WPI_MotorControlSetOutput.vi"("Output"=w342, "MotorControlDevRef"=w357) -> ("error out"=w350:errorcluster, "MotorControlDevRef"=w351:T2)  [unwired: 7 in, 1 out]
          n228 = call <vilib>:"WPI_MotorControlSetOutput.vi"("Output"=w341, "MotorControlDevRef"=w356) -> ("error out"=w348:errorcluster, "MotorControlDevRef"=w349:T2)  [unwired: 7 in, 1 out]
          n229 = call <vilib>:"WPI_MotorControlSetOutput.vi"("Output"=w342, "MotorControlDevRef"=w358) -> ("error out"=w352:errorcluster, "MotorControlDevRef"=w353:T2)  [unwired: 7 in, 1 out]
          n230 = call <vilib>:"Spark MAX Set Idle Mode.vi"("error in (no error)"=w352, "Idle Mode"=w345, "MotorControlDeviceRef in"=w353) -> ()  [unwired: 7 in, 2 out]
          n231 = call <vilib>:"Spark MAX Set Idle Mode.vi"("error in (no error)"=w346, "Idle Mode"=w345, "MotorControlDeviceRef in"=w347) -> ()  [unwired: 7 in, 2 out]
          n232 = call <vilib>:"Spark MAX Set Idle Mode.vi"("error in (no error)"=w350, "Idle Mode"=w345, "MotorControlDeviceRef in"=w351) -> ()  [unwired: 7 in, 2 out]
          n233 = call <vilib>:"Spark MAX Set Idle Mode.vi"("error in (no error)"=w348, "Idle Mode"=w345, "MotorControlDeviceRef in"=w349) -> ()  [unwired: 7 in, 2 out]
          n234 = Wait (ms)(milliseconds to wait=u32 1) -> ()  [unwired: 1 out]
        }
      }
    }
    n235 = Wait (ms)(milliseconds to wait=u32 1) -> ()  [unwired: 1 out]
  }
  n236 = disable-structure shown="Disabled" {
    frame Disabled {
      n237 = call <vilib>:"WPI_JoystickRefNum Registry Get.vi"("refnum name"="Joystick 0") -> ("JoystickDevRef"=w366:T8)  [unwired: 1 in, 9 out]
      n238 = call <vilib>:"WPI_JoystickRefNum Registry Get.vi"("refnum name"="Joystick 1") -> ("JoystickDevRef"=w364:T8)  [unwired: 1 in, 9 out]
      n239 = while {
        tunnel: w366 -> [w396]
        shift-right: [w380] -> _
        shift-left: _ -> [w385]
        tunnel: w364 -> [w370]
        stop <- FALSE stop-if-true
        n240 = global read "Robot Global Data.vi" "CUBE ITK SUP"() -> (w383:bool)
        n241 = global read "Robot Global Data.vi" "CUBE ITK INF"() -> (w384:bool)
        n242 = global read "Robot Global Data.vi" "LIME ALINHAMENTO"() -> (w398:bool)
        n243 = Divide(x=500.0 ("y"), y=5.0) -> (x/y=w387:dbl)
        n244 = global read "TOGGLE GLOBAL.vi" "TOGGLE 3"() -> (w373:bool)
        n245 = global read "Robot Global Data.vi" "AUTO_FREIO"() -> (w371:bool)
        n246 = Increment(x=w385) -> (x+1=w392:dbl)
        n247 = global read "TOGGLE GLOBAL.vi" "TOGGLE 6"() -> (w397:bool)
        n248 = Wait (ms)(milliseconds to wait=u32 5) -> ()  [unwired: 1 out]
        n249 = Less Or Equal?(x=w385, y=w387) -> (x <= y?=w376:bool)
        n250 = Not(x=w373) -> (.not. x?=w372:bool)
        n251 = Or(x=w384, y=w383) -> (x .or. y?=w382:bool)
        n252 = Or(x=w371, y=w372) -> (x .or. y?=w369:bool)
        n253 = Or(x=w398, y=w397) -> (x .or. y?=w395:bool)
        n254 = Select(t=w392, s=w382, f=0.0) -> (s? t:f=w381:dbl)
        n255 = Select(t=0.3, s=w395, f=0.0) -> (s? t:f=w378:dbl)
        n256 = Select(t=w381, s=w376, f=0.0) -> (s? t:f=w380:dbl)
        n257 = Select(t=1.0, s=w376, f=w378) -> (s? t:f=w374:dbl)
        n258 = Select(t=1.0, s=w369, f=w374) -> (s? t:f=w375:dbl)
        n259 = call <vilib>:"WPI_JoystickSetOutputs.vi"("Right Rumble"=w374, "Left Rumble"=w374, "JoystickDevRef"=w396) -> ()  [unwired: 7 in, 2 out]
        n260 = call <vilib>:"WPI_JoystickSetOutputs.vi"("Right Rumble"=w375, "Left Rumble"=w375, "JoystickDevRef"=w370) -> ()  [unwired: 7 in, 2 out]
      }
    }
    frame Enabled {
    }
  }
  n261 = while {
    stop <- FALSE stop-if-true
    n262 = global read "Robot Global Data.vi" "BTN A"() -> (w405:bool)
    n263 = global read "Robot Global Data.vi" "BTN Y"() -> (w401:bool)
    n264 = global read "Robot Global Data.vi" "ALT"() -> (w399:bool)
    n265 = call "TOGGLE 1.vi"("CLK"=w405) -> ()  [unwired: 5 in]
    n266 = call "TOGGLE 4.vi"("CLK"=w399) -> ()  [unwired: 5 in]
    n267 = call "TOGGLE 2.vi"("CLK"=w401) -> ()  [unwired: 5 in]
    n268 = global read "Robot Global Data.vi" "BTN X"() -> (w400:bool)
    n269 = global read "Robot Global Data.vi" "BTN B"() -> (w402:bool)
    n270 = Wait (ms)(milliseconds to wait=u32 5) -> ()  [unwired: 1 out]
    n271 = call "TOGGLE 6.vi"("CLK"=w402) -> ()  [unwired: 5 in]
    n272 = call "TOGGLE 3.vi"("CLK"=w400) -> ()  [unwired: 5 in]
  }
  n273 = call <vilib>:"WPI_MotorControlRefNum Registry Get.vi"("refnum name"="ITK MVT SUP") -> ("MotorControlDevRef"=w10:T2)  [unwired: 9 in, 1 out]
  n274 = call <vilib>:"WPI_DigitalInputRefNum Registry Get.vi"("refnum name"="FC ITK MVT SUP") -> ("DigitalInputDevRef"=w12:T10)  [unwired: 9 in, 1 out]
  n275 = call <vilib>:"WPI_MotorControlRefNum Registry Get.vi"("refnum name"="ITK CLT SUP") -> ("MotorControlDevRef"=w8:T2)  [unwired: 9 in, 1 out]
  n276 = call <vilib>:"WPI_EncoderRefNum Registry Get.vi"("refnum name"="CHASSI MD ENC") -> ("EncoderDevRef"=w25:T11)  [unwired: 9 in, 1 out]
  n277 = call <vilib>:"WPI_MotorControlRefNum Registry Get.vi"("refnum name"="ITK MVT INF") -> ("MotorControlDevRef"=w21:T2)  [unwired: 9 in, 1 out]
  n278 = call <vilib>:"WPI_DigitalInputRefNum Registry Get.vi"("refnum name"="FC ITK MVT INF") -> ("DigitalInputDevRef"=w19:T10)  [unwired: 9 in, 1 out]
  n279 = call <vilib>:"CTRE_PigeonIMU_RefNumRegistryGet.vi"("refnum name"="CHASSI PGN") -> ("PigeonIMUDevRef"=w23:T15)  [unwired: 9 in, 1 out]
  n280 = call <vilib>:"WPI_MotorControlRefNum Registry Get.vi"("refnum name"="ITK CLT INF") -> ("MotorControlDevRef"=w17:T2)  [unwired: 9 in, 1 out]
  n281 = while {
    tunnel: w25 -> [w443]
    tunnel: w23 -> [w435]
    tunnel: w21 -> [w433]
    tunnel: w19 -> [w432]
    tunnel: w17 -> [w424]
    tunnel: w10 -> [w412]
    tunnel: w12 -> [w413]
    tunnel: w8 -> [w409]
    stop <- FALSE stop-if-true
    w408 = 20  # Samples
    w420 = 40  # Samples
    w426 = 20  # Samples
    n282 = global read "Robot Global Data.vi" "CHASSI MD ENC RST"() -> (w440:bool)
    n283 = call-poly <vilib>:"CTRE_Phoenix_Pigeon2_GetStatus.vi"("PigeonIMUDevRef"=w435) -> ("Yaw Pitch Roll"=w438:cluster{"Yaw":dbl, "Pitch":dbl, "Roll":dbl})  [unwired: 8 in, 2 out]
    "Yaw Pitch Roll" <- w438
    n284 = call <vilib>:"Spark MAX Get Supply Current.vi"("MotorControlDevRef in"=w409) -> ("Current"=w406:dbl)  [unwired: 7 in, 3 out]
    "CORRENTE ITK INF 2" <- w406
    n285 = call <vilib>:"Spark MAX Get Supply Current.vi"("MotorControlDevRef in"=w424) -> ("Current"=w428:dbl)  [unwired: 7 in, 3 out]
    "CORRENTE ITK INF" <- w428
    n286 = call <vilib>:"WPI_DigitalInputGetValue.vi"("DigitalInputDevRef"=w413) -> ("Value"=w416:bool)  [unwired: 8 in, 2 out]
    n287 = call <vilib>:"WPI_DigitalInputGetValue.vi"("DigitalInputDevRef"=w432) -> ("Value"=w429:bool)  [unwired: 8 in, 2 out]
    n288 = Or(x=w440, y="RST MECE") -> (x .or. y?=w441:bool)
    n289 = Or(x="RST MGVT SUP", y=w416) -> (x .or. y?=w414:bool)
    n290 = Or(x="RST MGVT", y=w429) -> (x .or. y?=w431:bool)
    n291 = Unbundle By Name(w438) -> ("Yaw"=w418:dbl, "Pitch"=w437:dbl, "Roll"=w436:dbl)
    n292 = case shown="True" w441 {
      tunnel: w443 -> [_ w450]
      frame False {
      }
      frame True {
        n293 = call <vilib>:"WPI_EncoderReset.vi"("EncoderDevRef"=w450) -> ()  [unwired: 9 in, 2 out]
      }
    }
    n294 = case shown="True" w414 {
      tunnel: w412 -> [_ w444]
      frame False {
      }
      frame True {
        n295 = call <vilib>:"Spark MAX Set Sensor Position.vi"("Position"=0.0, "MotorControlDeviceRef"=w444) -> ()  [unwired: 8 in, 2 out]
      }
    }
    n296 = case shown="True" w431 {
      tunnel: w433 -> [_ w446]
      frame False {
      }
      frame True {
        n297 = call <vilib>:"Spark MAX Set Sensor Position.vi"("Position"=0.0, "MotorControlDeviceRef"=w446) -> ()  [unwired: 8 in, 2 out]
      }
    }
    n298 = call <vilib>:"WPI_EncoderGet.vi"("EncoderDevRef"=w443) -> ("Distance"=w422:dbl)  [unwired: 5 in, 5 out]
    "DISTANCE CHASSI(m)" <- w422
    n299 = global read "Robot Global Data.vi" "ACL YAW RST"() -> (w421:bool)
    n300 = call <vilib>:"Spark MAX Get Sensor Position.vi"("MotorControlDevRef in"=w412) -> ("Sensor Position"=w411:dbl)  [unwired: 7 in, 3 out]
    "DISTANCE ITK MVT SUP" <- w411
    n301 = call <vilib>:"Spark MAX Get Sensor Position.vi"("MotorControlDevRef in"=w433) -> ("Sensor Position"=w434:dbl)  [unwired: 7 in, 3 out]
    "DISTANCE ITK MVT" <- w434
    n302 = global write "Robot Global Data.vi" "ACL PITCH"(w437) -> ()
    n303 = global write "Robot Global Data.vi" "ACL ROLL"(w436) -> ()
    n304 = call <vilib>:"LinearFilter_Execute.vi"("Samples"=w408, "Filter Type"=T17."Moving Average", "Input"=w406) -> ("Output"=→"CORRENTE INTAKE 3":dbl)  [unwired: 7 in, 1 out]
    n305 = call <vilib>:"LinearFilter_Execute.vi"("Samples"=w426, "Filter Type"=T17."Moving Average", "Input"=w428) -> ("Output"=→"CORRENTE INTAKE 2":dbl)  [unwired: 7 in, 1 out]
    n306 = global write "Robot Global Data.vi" "ITK MVT SUP ENC"(w411) -> ()
    n307 = call <vilib>:"LinearFilter_Execute.vi"("Samples"=w420, "Filter Type"=T17."Moving Average", "Input"=w418) -> ("Output"=w417:dbl)  [unwired: 7 in, 1 out]
    n308 = global write "Robot Global Data.vi" "CHASSI MD ENC"(w422) -> ()
    n309 = global write "Robot Global Data.vi" "ITK MVT INF ENC"(w434) -> ()
    n310 = global write "Robot Global Data.vi" "ITK SUP CLT I"(w406) -> ()
    n311 = global write "Robot Global Data.vi" "ITK INF CLT I"(w428) -> ()
    n312 = global write "Robot Global Data.vi" "ITK SUP MVT FC"(w416) -> ()
    n313 = global write "Robot Global Data.vi" "ITK INF MVT FC"(w429) -> ()
    n314 = Wait (ms)(milliseconds to wait=u32 1) -> ()  [unwired: 1 out]
    n315 = global write "Robot Global Data.vi" "ACL YAW"(w417) -> ()
    n316 = case shown="True" w421 {
      tunnel: w435 -> [_ w448]
      frame False {
      }
      frame True {
        n317 = call <vilib>:"CTRE_PigeonIMU_SetYaw.vi"("Value"=0.0, "PigeonIMUDevRef"=w448) -> ()  [unwired: 8 in, 2 out]
      }
    }
  }
  n318 = while {
    stop <- FALSE stop-if-true
    # "3 = CUBE"
    # "1 =  GRID"
    n319 = Wait (ms)(milliseconds to wait=u32 10) -> ()  [unwired: 1 out]
    n320 = call-poly <vilib>:"NT Read Value.vi"("name"="/limelight/tx" ("Name")) -> ("value"=w455:dbl)  [unwired: 8 in, 2 out]
    "tx" <- w455
    n321 = call-poly <vilib>:"NT Read Value.vi"("name"="/limelight\\ty" ("Name")) -> ("value"=→"ty":dbl)  [unwired: 8 in, 2 out]
    n322 = call-poly <vilib>:"NT Read Value.vi"("name"="/limelight/ta" ("Name")) -> ("value"=→"ta":dbl)  [unwired: 8 in, 2 out]
    n323 = call-poly <vilib>:"NT Read Value.vi"("name"="/limelight/ts" ("Name")) -> ("value"=→"ts":dbl)  [unwired: 8 in, 2 out]
    n324 = global write "Robot Global Data.vi" "LIME_TX"(w455) -> ()
    n325 = global read "Robot Global Data.vi" "LIME_LED"() -> (w453:dbl)
    n326 = global read "Robot Global Data.vi" "PIPELINE SLC"() -> (w454:dbl)
    n327 = call-poly <vilib>:"NT Write Value.vi"("value"=w453, "name"="/limelight/ledMode" ("Name")) -> ()  [unwired: 9 in, 1 out]
    n328 = call-poly <vilib>:"NT Write Value.vi"("value"=w454, "name"="/limelight/pipeline" ("Name")) -> ()  [unwired: 9 in, 1 out]
  }
  n329 = call <vilib>:"WPI_JoystickRefNum Registry Get.vi"("refnum name"="Joystick 0") -> ("JoystickDevRef"=w1:T8)  [unwired: 1 in, 9 out]
  n330 = call <vilib>:"WPI_JoystickRefNum Registry Get.vi"("refnum name"="Joystick 1") -> ("JoystickDevRef"=w2:T8)  [unwired: 1 in, 9 out]
  n331 = while {
    shift-right: [w468] -> _
    shift-left: _ -> [w467]
    tunnel: w2 -> [w466]
    tunnel: w1 -> [w465]
    stop <- FALSE stop-if-true
    n332 = call <vilib>:"WPI_DriverStationGetModeAndStatus.vi"() -> ("Robot Mode"=w469:T18)  [unwired: 10 in, 1 out]
    n333 = Wait (ms)(milliseconds to wait=u32 5) -> ()  [unwired: 1 out]
    n334 = Equal?(x=w469, y=WPI_DriverStationRobotMode2."Disconnected" ("Robot Mode")) -> (x = y?=w470:bool)
    n335 = case shown="True" w470 {
      tunnel: w469 -> [_ _]
      tunnel: [w477 _] -> w468
      tunnel: w467 -> [w476 _]
      tunnel: w466 -> [w475 _]
      tunnel: w465 -> [w474 _]
      frame False {
        n336 = call <vilib>:"WPI_DriverStationGetModeAndStatus.vi"() -> ("Robot Mode"=w479:T18)  [unwired: 10 in, 1 out]
        n337 = Equal?(x=w479, y=WPI_DriverStationRobotMode2."Teleop Enabled" ("Robot Mode")) -> (x = y?=w478:bool)
        n338 = case shown="True" w478 {
          tunnel: [_ w489] -> w477
          tunnel: w476 -> [_ w494]
          tunnel: w475 -> [_ w498]
          tunnel: w474 -> [_ w497]
          frame False {
            n339 = disable-structure shown="Disabled" {
              frame Disabled {
                n340 = global write "Robot Global Data.vi" "LIME_LED"(1.0 ("LIME_LED")) -> ()
              }
              frame Enabled {
              }
            }
            n341 = global write "Robot Global Data.vi" "CHASSI BREAK"(FALSE ("CHASSI BREAK")) -> ()
            n342 = call-poly <vilib>:"NT Read Value.vi"("default value"=1.0, "name"="LimeLight_LED") -> ("value"=w481:dbl)  [unwired: 7 in, 2 out]
            n343 = global write "Robot Global Data.vi" "LIME_LED"(w481) -> ()
          }
          frame True {
            n344 = global write "Robot Global Data.vi" "CHASSI BREAK"(TRUE ("CHASSI BREAK")) -> ()
            n345 = disable-structure shown="Disabled" {
              frame Disabled {
                n346 = global read "TOGGLE GLOBAL.vi" "TOGGLE 6"() -> (w529:bool)
                n347 = Select(t=0.0, s=w529, f=1.0) -> (s? t:f=w532:dbl)
                n348 = global write "Robot Global Data.vi" "LIME_LED"(w532) -> ()
              }
              frame Enabled {
              }
            }
            n349 = Divide(x=1000.0 ("y"), y=5.0) -> (x/y=w490:dbl)
            n350 = global read "Robot Global Data.vi" "CUBE ITK SUP"() -> (w507:bool)
            n351 = global read "Robot Global Data.vi" "CUBE ITK INF"() -> (w508:bool)
            n352 = global read "Robot Global Data.vi" "LIME ALINHAMENTO"() -> (w518:bool)
            n353 = Divide(x=10.0 ("y"), y=5.0) -> (x/y=w491:dbl)
            n354 = call-poly <vilib>:"NT Read Value.vi"("default value"=0.2, "name"="AUX1") -> ("value"=w527:dbl)  [unwired: 7 in, 2 out]
            n355 = call-poly <vilib>:"NT Read Value.vi"("default value"=0.13, "name"="AUX2") -> ("value"=w522:dbl)  [unwired: 7 in, 2 out]
            n356 = call-poly <vilib>:"NT Read Value.vi"("default value"=3.0, "name"="AUX3") -> ("value"=w519:dbl)  [unwired: 7 in, 2 out]
            n357 = global read "TOGGLE GLOBAL.vi" "TOGGLE 3"() -> (w496:bool)
            n358 = global read "Robot Global Data.vi" "AUTO_FREIO"() -> (w501:bool)
            n359 = Increment(x=w494) -> (x+1=w513:dbl)
            n360 = global read "TOGGLE GLOBAL.vi" "TOGGLE 6"() -> (w517:bool)
            n361 = In Range and Coerce(upper limit=w490, x=w494, lower limit=w491) -> (In Range?=w495:bool)  [unwired: 1 out]
            n362 = global write "Robot Global Data.vi" "LIME_AJUSTE_BRUTO"(w527) -> ()
            n363 = global write "Robot Global Data.vi" "LIME_AJUSTE_FINO"(w522) -> ()
            n364 = global write "Robot Global Data.vi" "PIPELINE SLC"(w519) -> ()
            n365 = Or(x=w508, y=w507) -> (x .or. y?=w506:bool)
            n366 = Or(x=w501, y=w496) -> (x .or. y?=w500:bool)
            n367 = Or(x=w518, y=w517) -> (x .or. y?=w516:bool)
            n368 = Select(t=w513, s=w506, f=0.0) -> (s? t:f=w489:dbl)
            n369 = Select(t=0.3, s=w516, f=0.0) -> (s? t:f=w505:dbl)
            n370 = Select(t=1.0, s=w495, f=w505) -> (s? t:f=w502:dbl)
            n371 = Select(t=1.0, s=w500, f=w502) -> (s? t:f=w503:dbl)
            n372 = call-poly <vilib>:"NT Read Value.vi"("default value"=1.0, "name"="LimeLight_LED") -> ("value"=w486:dbl)  [unwired: 7 in, 2 out]
            n373 = call <vilib>:"WPI_JoystickSetOutputs.vi"("Right Rumble"=w502, "Left Rumble"=w502, "JoystickDevRef"=w497) -> ()  [unwired: 7 in, 2 out]
            n374 = call <vilib>:"WPI_JoystickSetOutputs.vi"("Right Rumble"=w503, "Left Rumble"=w503, "JoystickDevRef"=w498) -> ()  [unwired: 7 in, 2 out]
            n375 = global write "Robot Global Data.vi" "LIME_LED"(w486) -> ()
            n376 = Wait (ms)(milliseconds to wait=u32 5) -> ()  [unwired: 1 out]
          }
        }
      }
      frame True {
        n377 = global write "Robot Global Data.vi" "CHASSI BREAK"(FALSE ("CHASSI BREAK")) -> ()
        n378 = global write "Robot Global Data.vi" "LIME_LED"(1.0 ("LIME_LED")) -> ()
      }
    }
  }
  n379 = disable-structure shown="Disabled" {
    frame Disabled {
      n380 = call-poly <vilib>:"NT Write Value.vi"("value"="AUX 13", "name"="AUX13") -> ()  [unwired: 9 in, 1 out]
      n381 = call-poly <vilib>:"NT Write Value.vi"("value"="Velocidade", "name"="Velocidade") -> ()  [unwired: 9 in, 1 out]
      n382 = call-poly <vilib>:"NT Write Value.vi"("value"="AUX 14", "name"="AUX14") -> ()  [unwired: 9 in, 1 out]
      n383 = call-poly <vilib>:"NT Write Value.vi"("value"="AUX 7", "name"="AUX7") -> ()  [unwired: 9 in, 1 out]
      n384 = call-poly <vilib>:"NT Write Value.vi"("value"="AUX 5", "name"="AUX5") -> ()  [unwired: 9 in, 1 out]
      n385 = call-poly <vilib>:"NT Write Value.vi"("value"="AUX 1", "name"="AUX1") -> ()  [unwired: 9 in, 1 out]
      n386 = call-poly <vilib>:"NT Write Value.vi"("value"="AUX 11", "name"="AUX11") -> ()  [unwired: 9 in, 1 out]
      n387 = call-poly <vilib>:"NT Write Value.vi"("value"="AUX 3", "name"="AUX3") -> ()  [unwired: 9 in, 1 out]
      n388 = call-poly <vilib>:"NT Write Value.vi"("value"="AUX 9", "name"="AUX9") -> ()  [unwired: 9 in, 1 out]
      n389 = call-poly <vilib>:"NT Write Value.vi"("value"="AUX 8", "name"="AUX8") -> ()  [unwired: 9 in, 1 out]
      n390 = call-poly <vilib>:"NT Write Value.vi"("value"="AUX 2", "name"="AUX2") -> ()  [unwired: 9 in, 1 out]
      n391 = call-poly <vilib>:"NT Write Value.vi"("value"="AUX 6", "name"="AUX6") -> ()  [unwired: 9 in, 1 out]
      n392 = call-poly <vilib>:"NT Write Value.vi"("value"="AUX 4", "name"="AUX4") -> ()  [unwired: 9 in, 1 out]
      n393 = call-poly <vilib>:"NT Write Value.vi"("value"="AUX 12", "name"="AUX12") -> ()  [unwired: 9 in, 1 out]
      n394 = call-poly <vilib>:"NT Write Value.vi"("value"="AUX 10", "name"="AUX10") -> ()  [unwired: 9 in, 1 out]
    }
    frame Enabled {
    }
  }
